vi "run.list.vi"(8 "error in":errorcluster, 11 "Client in":refnum<class "Client.lvclass">) -> (0 "error out":errorcluster, 3 "Client out":refnum<class "Client.lvclass">)   [LabVIEW 2020, in "Client.lvclass"]
doc: "Lists all runs, newest first, and returns a handle list of matches."
uses:
  Client.lvclass
  Client.lvclass/Client.ctl
  client.lvlib
panel:
  out "out_list out":i32
  out "out_count out":u32
  in  "out_list":i32
  in  "out_count":u32
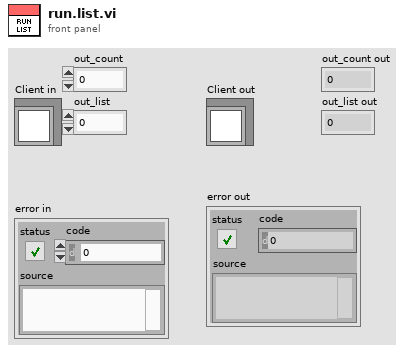
[diagram p1: front panel]
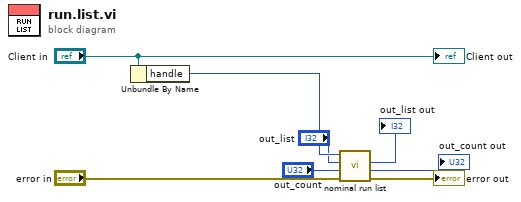
[diagram p0: block diagram]
diagram:
  n1 = Unbundle By Name("Client in") -> ("handle"=w6:i32)
  n2 = call "nominal run list.vi"("error in (no error)"="error in", "out_count"="out_count", "out_list"="out_list", "client"=w6) -> ("error out"=→"error out":errorcluster, "out_count out"=→"out_count out":u32, "out_list out"=→"out_list out":i32)  [unwired: 4 in, 1 out]
  "Client out" <- "Client in"
